vi "Insert Brower Panel.vi"(8 "error in (no error)":errorcluster, 11 "Panel Manager Controller.lvclass":refnum<class "Panel Manager Controller.lvclass">) -> (0 "error out":errorcluster, 3 "Panel Manager Controller.lvclass":refnum<class "Panel Manager Controller.lvclass">)   [LabVIEW 2015, in "Panel Manager Controller.lvclass"]
uses:
  Panel Manager Controller.lvclass
  Panel Manager Controller.lvclass/Panel Manager Controller.ctl
  Browers/Brower Controller/Browers Controller.lvclass
  Panel View/Panel View.lvclass/Panel View.ctl
  Browers/Browers Controller Messages/Insert Brower Panel in Subpanel Msg/Insert Brower Panel in Subpanel Msg.lvclass/Insert Brower Panel in Subpanel Msg.ctl
  <vilib>/ActorFramework/Message Enqueuer/Message Enqueuer.lvclass/Message Enqueuer.ctl
  <vilib>/ActorFramework/Message Enqueuer/Enqueue.vi
  <vilib>/ActorFramework/Message Priority Queue/Priority Enqueue.vi
  Browers/Browers Controller Messages/Insert Brower Panel in Subpanel Msg/Insert Brower Panel in Subpanel Msg.lvclass
  <vilib>/ActorFramework/Actor/Actor.lvclass
  Panel View/Panel View.lvclass
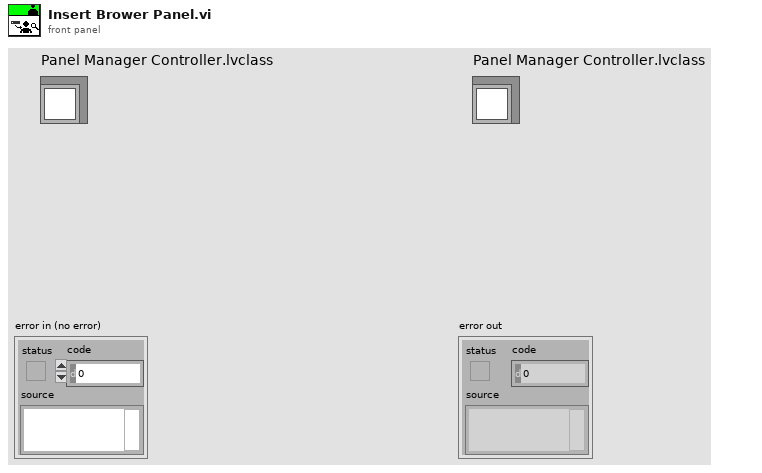
[diagram p1: front panel]
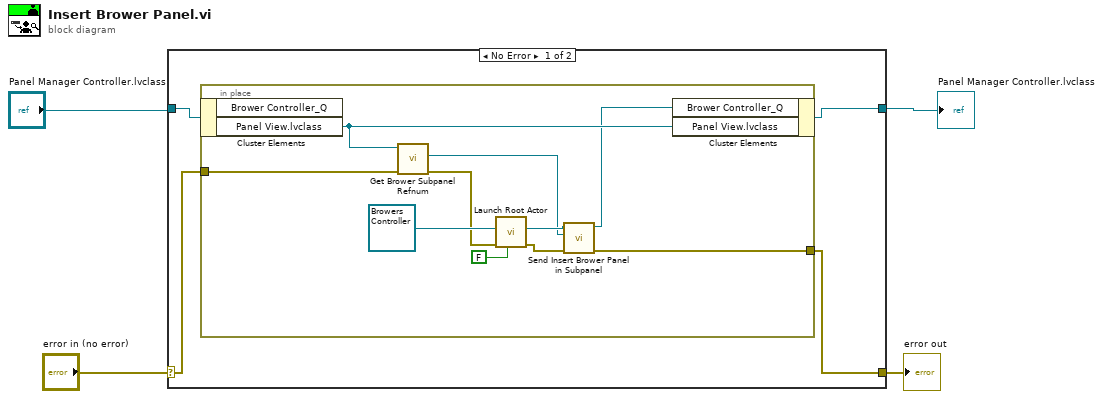
[diagram p0: block diagram]
diagram:
  n1 = case shown="No Error" "error in (no error)" {
    selector: "error in (no error)" -> [w8 w20]
    tunnel: [w5 w20] -> w3
    tunnel: [w6 w19] -> w1
    tunnel: "Panel Manager Controller.lvclass" -> [w7 w19]
    frame No Error {
      n2 = in-place {
        in-place-border: w8 -> [w18]
        in-place-border: [w10] -> w5
        n3 = in-place-cluster #1(w7) -> ("Panel View.lvclass"=w15:refnum<class "Panel View.lvclass">)  [unwired: 1 out]
        n4 = call "Get Brower Subpanel Refnum.vi"("error in (no error)"=w18, "Panel View in"=w15) -> ("error out"=w16:errorcluster, "Brower Subpanel Refnum"=w13:refnum<vi>)  [unwired: 7 in, 1 out]
        n5 = call <vilib>:"Launch Root Actor.vi"("Open Actor Core front panel? (F)"=FALSE, "error in (no error)"=w16, "Actor"=refnum<class "Browers Controller.lvclass"> refnum ("Browers")) -> ("error out"=w12:errorcluster, "Actor's Enqueuer"=w14:refnum<class "Message Enqueuer.lvclass">)  [unwired: 7 in]
        n6 = call "Send Insert Brower Panel in Subpanel.vi"("error in (no error)"=w12, "Brower Subpanel Refnum"=w13, "Message Enqueuer"=w14) -> ("error out"=w10:errorcluster, "Message Enqueuer out"=w11:refnum<class "Message Enqueuer.lvclass">)  [unwired: 7 in]
        n7 = in-place-cluster #1("Brower Controller_Q"=w11, "Panel View.lvclass"=w15) -> (w6:refnum<class "Panel Manager Controller.lvclass">)
      }
    }
    frame Error {
    }
  }
  "error out" <- w3
  "Panel Manager Controller.lvclass" <- w1
